vi "parseLaserScan.vi"(4 "error in":errorcluster, 7 "msg in":string) -> (0 "error out":errorcluster, 1 "Bearing Array":dbl[](array[numeric]), 2 "Range Array":sgl[](array[numeric]), 3 "Scan Details":T1)   [LabVIEW 2014]
doc: "Parses a message into a range"
uses:
  <vilib>/Tufts CEEO ROS for LabVIEW Software/ROS/MessageParsing/std_msgs/subs/parse_float32_scalar.vi
panel:
  out "Numeric":i32
  out "x/y":sgl
  out "Size Bear.":i32
  out "size Range":i32
  out "msg out":string
  out "Header":T2
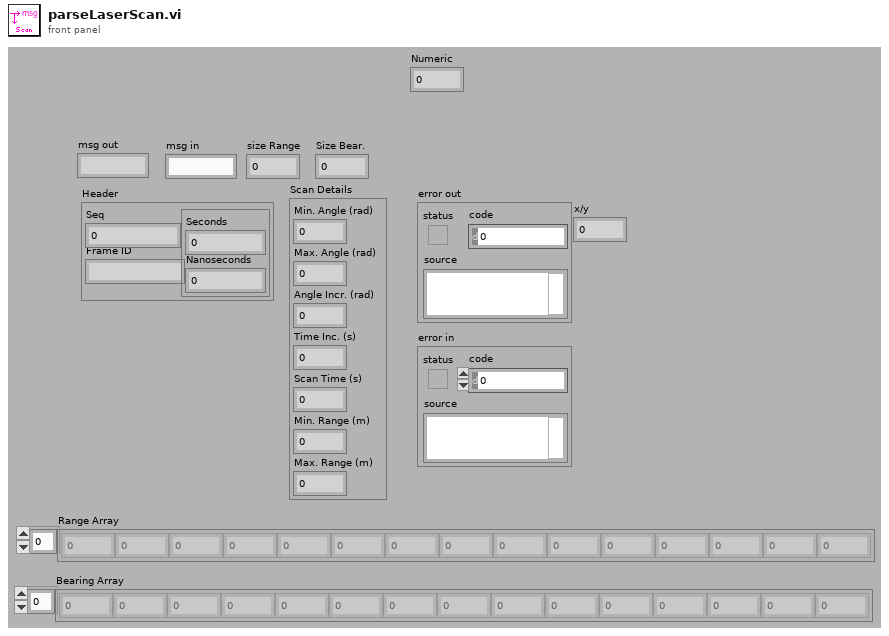
[diagram p1: front panel]
types:
  T1 = cluster{"Min. Angle (rad)":dbl, "Max. Angle (rad)":dbl, "Angle Incr. (rad)":dbl, "Time Inc. (s)":dbl, "Scan Time (s)":dbl, "Min. Range (m)":dbl, "Max. Range (m)":dbl}
  T2 = cluster{"Seq":u32, "Frame ID":string, cluster{"Seconds":i32, "Nanoseconds":i32}}
  T3 = cluster{"Seq":u32, "Frame ID":string, "Timestamp":cluster{"Seconds":i32, "Nanoseconds":i32}}
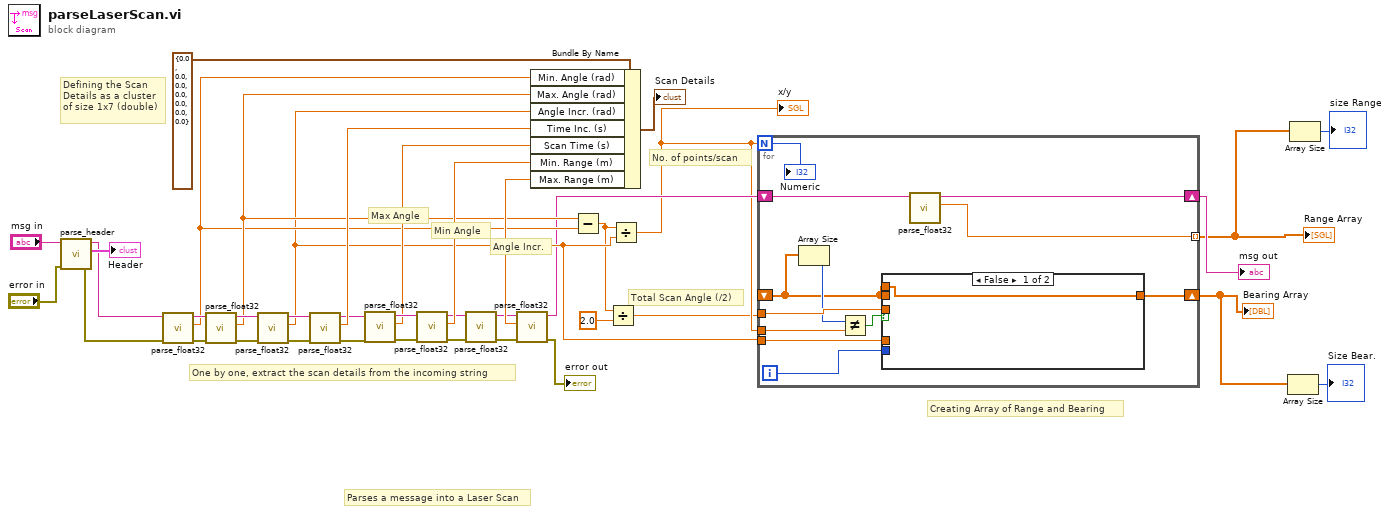
[diagram p0: block diagram]
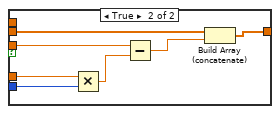
[diagram p2: hidden frame]
diagram:
  # "One by one, extract the scan details from the incoming string"
  # "Defining the Scan \nDetails as a cluster \nof size 1x7 (double)"
  # "Total Scan Angle (/2)"
  # "Angle Incr."
  # "Min Angle"
  # "Max Angle"
  # "No. of points/scan"
  # "Creating Array of Range and Bearing"
  # "Parses a message into a Laser Scan"
  n1 = call <vilib>:"parse_header.vi"("error in"="error in", "msg in"="msg in") -> ("error out"=w29:errorcluster, "Header"=→"Header":T3, "msg out"=w30:string)  [unwired: 3 in]
  n2 = call-poly <vilib>:"parse_float32.vi"("error in"=w29, "msg in"=w30) -> ("error out"=w37:errorcluster, "number"=w16:sgl, "msg out"=w38:string)  [unwired: 3 in]
  n3 = call-poly <vilib>:"parse_float32.vi"("error in"=w37, "msg in"=w38) -> ("error out"=w36:errorcluster, "number"=w17:sgl, "msg out"=w35:string)  [unwired: 3 in]
  n4 = call-poly <vilib>:"parse_float32.vi"("error in"=w36, "msg in"=w35) -> ("error out"=w33:errorcluster, "number"=w15:sgl, "msg out"=w34:string)  [unwired: 3 in]
  n5 = call-poly <vilib>:"parse_float32.vi"("error in"=w33, "msg in"=w34) -> ("error out"=w21:errorcluster, "number"=w27:sgl, "msg out"=w26:string)  [unwired: 3 in]
  n6 = call-poly <vilib>:"parse_float32.vi"("error in"=w21, "msg in"=w26) -> ("error out"=w20:errorcluster, "number"=w24:sgl, "msg out"=w25:string)  [unwired: 3 in]
  n7 = call-poly <vilib>:"parse_float32.vi"("error in"=w20, "msg in"=w25) -> ("error out"=w2:errorcluster, "number"=w23:sgl, "msg out"=w4:string)  [unwired: 3 in]
  n8 = call-poly <vilib>:"parse_float32.vi"("error in"=w2, "msg in"=w4) -> ("error out"=w1:errorcluster, "msg out"=w3:string)  [unwired: 3 in, 1 out]
  n9 = call-poly <vilib>:"parse_float32.vi"("error in"=w1, "msg in"=w3) -> ("error out"=→"error out":errorcluster, "number"=w22:sgl, "msg out"=w14:string)  [unwired: 3 in]
  n10 = Bundle By Name(cluster=T1 {"Min. Angle (rad)"=0.0, "Max. Angle (rad)"=0.0, "Angle Incr. (rad)"=0.0, "Time Inc. (s)"=0.0, "Scan Time (s)"=0.0, "Min. Range (m)"=0.0, "Max. Range (m)"=0.0}, "Min. Angle (rad)"=w16, "Max. Angle (rad)"=w17, "Angle Incr. (rad)"=w15, "Time Inc. (s)"=w27, "Scan Time (s)"=w24, "Min. Range (m)"=w23, "Max. Range (m)"=w22) -> (→"Scan Details":T1)
  n11 = Subtract(x=w17, y=w16) -> (x-y=w6:sgl)
  n12 = Divide(x=w6, y=2.0) -> (x/y=w5:dbl)
  n13 = Divide(x=w6, y=w15) -> (x/y=w8:sgl)
  "x/y" <- w8
  n14 = for {
    N: w8 -> [w40]
    tunnel: w15 -> [w50]
    shift-right: [w49] -> w9
    shift-left: _ -> [w41]
    shift-right: [w47] -> w13
    shift-left: w14 -> [w48]
    tunnel: [w46] -> w12 mode=indexing
    tunnel: w5 -> [w45]
    tunnel: w8 -> [w42]
    i -> [w51]
    n15 = Array Size(array=w41) -> (size(s)=w43:i32)
    n16 = Not Equal?(x=w43, y=w42) -> (x != y?=w44:bool)
    n17 = case shown="False" w44 {
      tunnel: w51 -> [_ w59]
      tunnel: w50 -> [_ w58]
      tunnel: [w52 w55] -> w49
      tunnel: w41 -> [_ w54]
      tunnel: w45 -> [_ w53]
      tunnel: w41 -> [w52 _]
      frame False {
      }
      frame True {
        n18 = Multiply(x=w58, y=w59) -> (x*y=w57:sgl)
        n19 = Subtract(x=w53, y=w57) -> (x-y=w56:dbl)
        n20 = Build Array (concatenate)(w54, w56) -> (w55:dbl[])
      }
    }
    n21 = call-poly <vilib>:"parse_float32.vi"("msg in"=w48) -> ("number"=w46:sgl, "msg out"=w47:string)  [unwired: 4 in, 1 out]
    "Numeric" <- w40
  }
  "Range Array" <- w12
  "Bearing Array" <- w9
  "msg out" <- w13
  n22 = Array Size(array=w9) -> (size(s)=→"Size Bear.":i32)
  n23 = Array Size(array=w12) -> (size(s)=→"size Range":i32)
